vi "odor manifold config to csv (top level vi).vi"() -> ()   [LabVIEW 2021]
uses:
  type-defs/odor and manifold config cluster (type def).ctl
  type-defs/manifold configuration cluster array (type def).ctl
  type-defs/manifold configuration cluster (type def).ctl
  type-defs/manifold selection.ctl
  type-defs/single port single odor cluster.ctl
  type-defs/port number (type def).ctl
  type-defs/odor selection (type def).ctl
  type-defs/odor color (type def).ctl
  type-defs/odor description array (type def).ctl
  type-defs/odor info cluster (type def).ctl
panel:
  out "csv lines out":string[](array[string])
  in  "interactive? (T)":bool=TRUE
  in  "odor manifold config in (none)":T1
  out "error out":errorcluster
  in  "error in (no error)":errorcluster
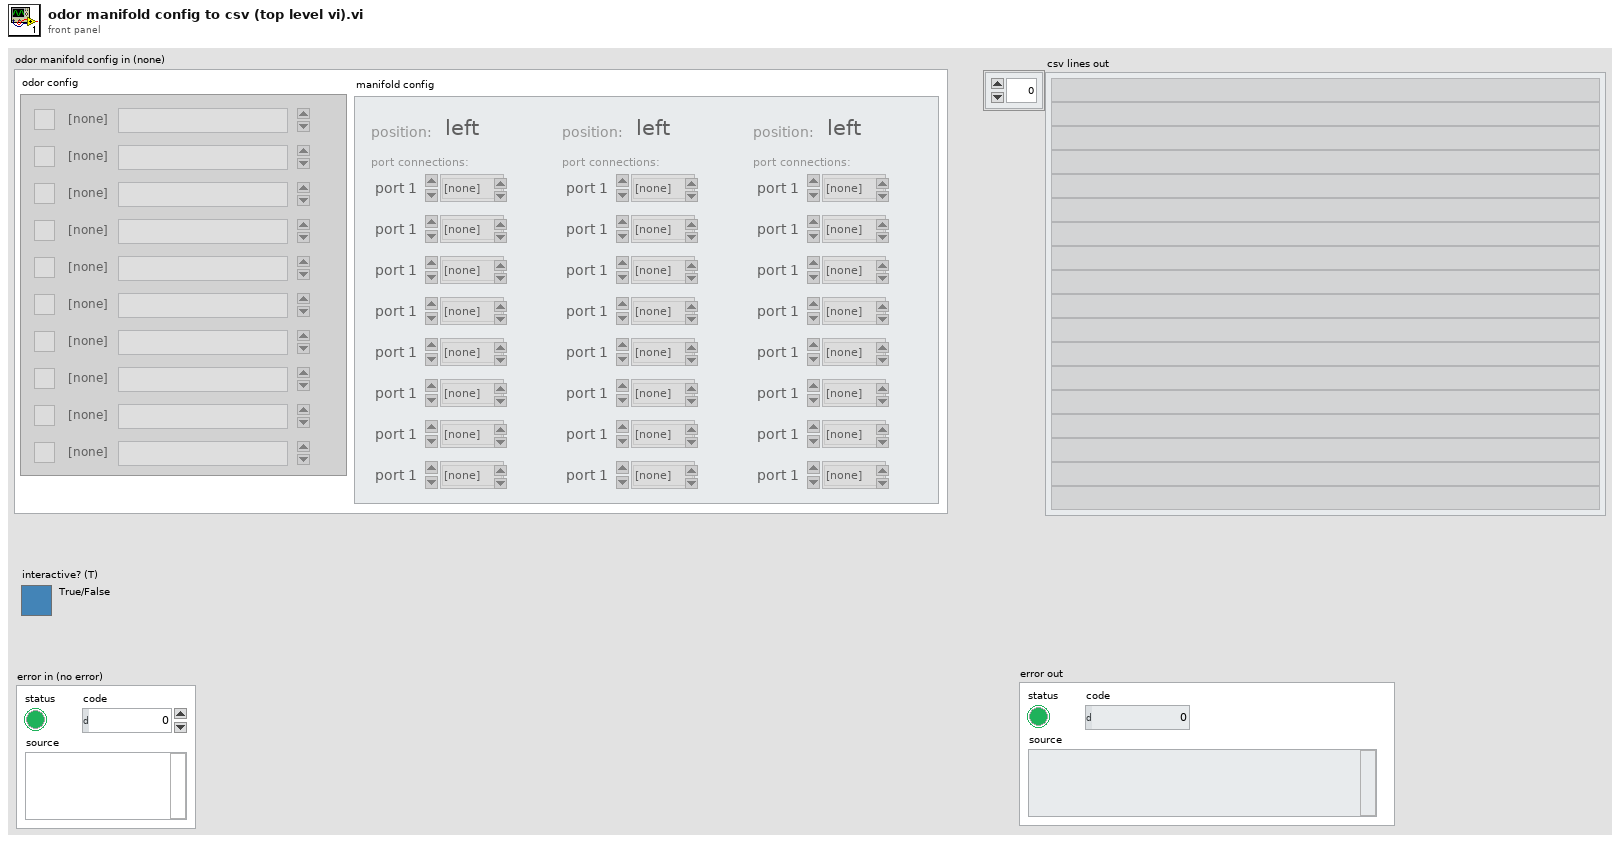
[diagram p1: front panel]
types:
  T1 = typedef "odor and manifold config cluster (type def).ctl" = cluster{"manifold config":T2, "odor config":T9}
  T2 = typedef "manifold configuration cluster array (type def).ctl" = T3[]
  T3 = typedef "manifold configuration cluster (type def).ctl" = cluster{"position:":T4, "port connections:":T5[]}
  T4 = typedef "manifold selection.ctl" = enum16{"left", "middle", "right"}
  T5 = typedef "single port single odor cluster.ctl" = cluster{"port number":T6, "connected odor":T7, "error":bool, "odor color":T8}
  T6 = typedef "port number (type def).ctl" = enum16{"port 1", "port 2", "port 3", "port 4", "port 5", "port 6", "port 7", "port 8"}
  T7 = typedef "odor selection (type def).ctl" = enum16{"[none]", "odor 1", "odor 2", "odor 3", "odor 4", "odor 5", "odor 6", "odor 7", "odor 8", "odor 9", "odor 10"}
  T8 = typedef "odor color (type def).ctl" = u16
  T9 = typedef "odor description array (type def).ctl" = T10[]
  T10 = typedef "odor info cluster (type def).ctl" = cluster{"odor channel":T7, "odor description":string, "odor color":T8, "odor channel active":bool}
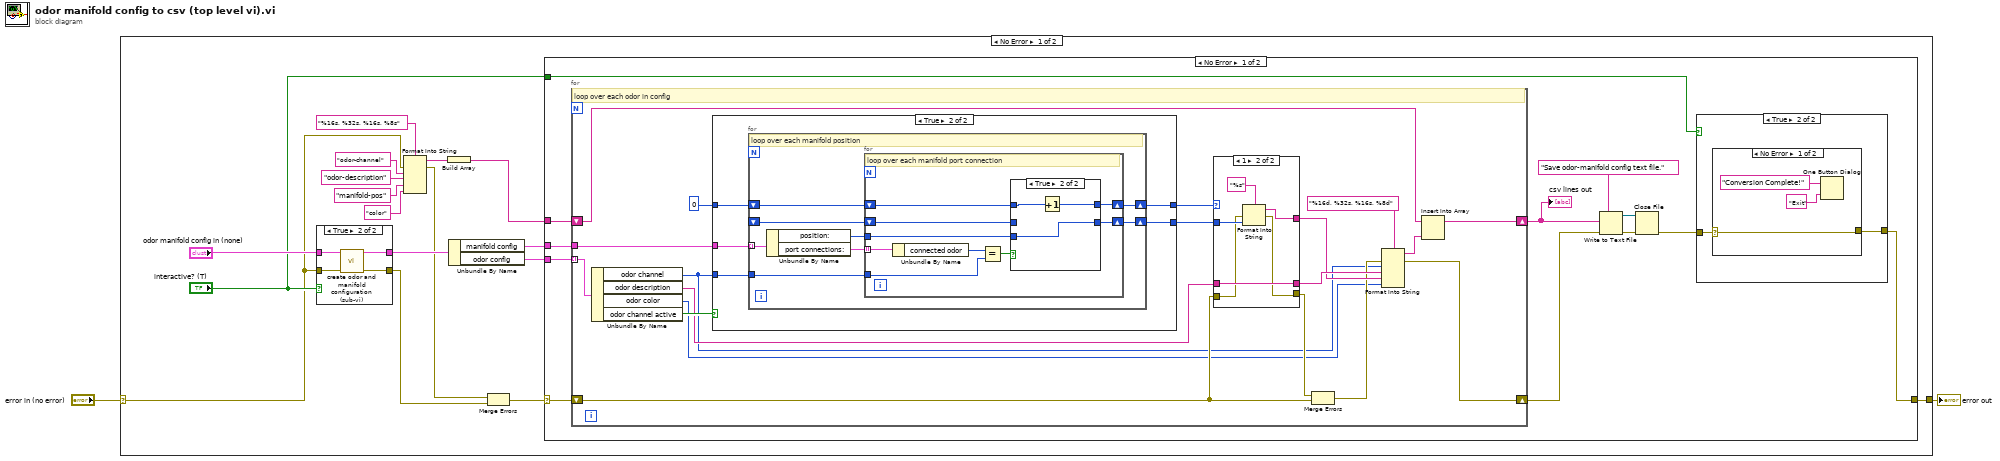
[diagram p0: block diagram]
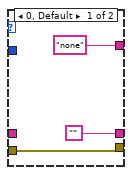
[diagram p5: hidden frame]
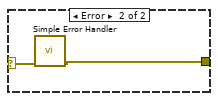
[diagram p7: hidden frame]
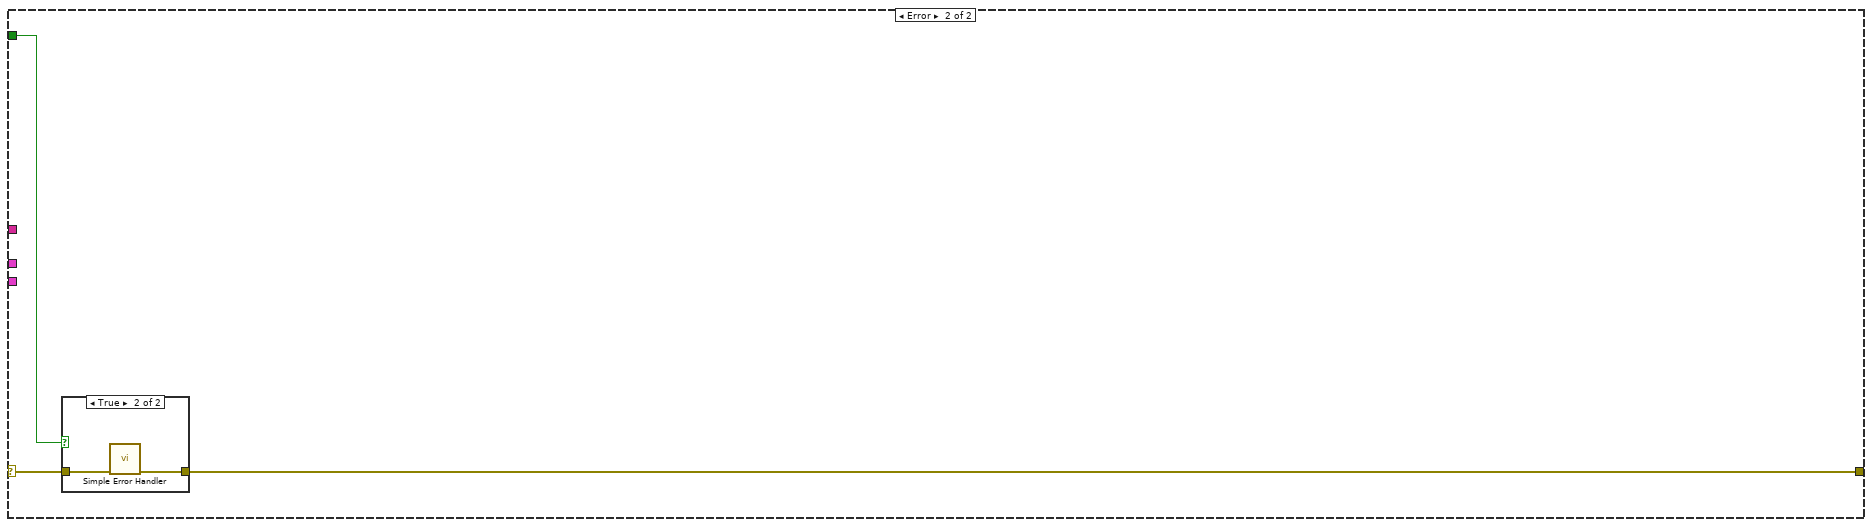
[diagram p8: hidden frame]
diagram:
  n1 = case shown="No Error" "error in (no error)" {
    selector: "error in (no error)" -> [w4 w108]
    tunnel: [w7 w108] -> w1
    frame No Error {
      n2 = case shown="True" "interactive? (T)" {
        tunnel: [w20 w25] -> w11
        tunnel: w4 -> [w21 w24]
        tunnel: [w21 w23] -> w8
        tunnel: "odor manifold config in (none)" -> [w20 w22]
        frame False {
        }
        frame True {
          n3 = call "create odor and manifold configuration (sub-vi).vi"("error in (no error)"=w24, "initial odor and manifold config (none)"=w22) -> ("error out"=w23:errorcluster, "odor and manifold config out"=w25:T1)  [unwired: 7 in, 1 out]
        }
      }
      n4 = Format Into String(format string="%16s, %32s, %16s, %8s", error in=w4, "odor-channel" ("input 1"), "odor-description" ("input 2"), "manifold-pos" ("input 3"), "color" ("input 4")) -> (resulting string=w16:string, error out=w9:errorcluster)  [unwired: 1 in]
      n5 = Build Array(w16) -> (w15:string[])
      n6 = Unbundle By Name(w11) -> ("manifold config"=w18:T2, "odor config"=w19:T9)
      n7 = Merge Errors(w9, w8) -> (w10:errorcluster)
      n8 = case shown="No Error" w10 {
        selector: w10 -> [w29 w104]
        tunnel: w19 -> [w37 _]
        tunnel: w18 -> [w36 _]
        tunnel: w15 -> [w35 _]
        tunnel: [w27 w103] -> w7
        tunnel: "interactive? (T)" -> [w26 w102]
        frame No Error {
          n9 = for {
            tunnel: w37 -> [w55] mode=indexing
            tunnel: w36 -> [w56]
            shift-right: [w46] -> w33
            shift-left: w35 -> [w45]
            shift-right: [w42] -> w30
            shift-left: w29 -> [w41]
            # "loop over each odor in config"
            n10 = Unbundle By Name(w55) -> ("odor channel"=w38:T7, "odor description"=w51:string, "odor color"=w39:T8, "odor channel active"=w54:bool)
            n11 = case shown="True" w54 {
              tunnel: w56 -> [_ w62]
              tunnel: w38 -> [_ w61]
              tunnel: [w57 w60] -> w53
              tunnel: [_ w59] -> w52
              tunnel: 0 -> [w57 w58]
              frame False {
              }
              frame True {
                n12 = for {
                  tunnel: w62 -> [w70] mode=indexing
                  tunnel: w61 -> [w68]
                  shift-right: [w66] -> w59
                  shift-left: _ -> [w65]
                  shift-right: [w63] -> w60
                  shift-left: w58 -> [w64]
                  # "loop over each manifold position"
                  n13 = Unbundle By Name(w70) -> ("position:"=w67:T4, "port connections:"=w69:T5[])
                  n14 = for {
                    tunnel: w69 -> [w79] mode=indexing
                    tunnel: w68 -> [w76]
                    tunnel: w67 -> [w75]
                    shift-right: [w74] -> w66
                    shift-left: w65 -> [w73]
                    shift-right: [w71] -> w63
                    shift-left: w64 -> [w72]
                    # "loop over each manifold port connection"
                    n15 = Unbundle By Name(w79) -> ("connected odor"=w78:T7)
                    n16 = Equal?(x=w78, y=w76) -> (x = y?=w77:bool)
                    n17 = case shown="True" w77 {
                      tunnel: w75 -> [_ w84]
                      tunnel: [w81 w84] -> w74
                      tunnel: w73 -> [w81 _]
                      tunnel: w72 -> [w80 w83]
                      tunnel: [w80 w82] -> w71
                      frame False {
                      }
                      frame True {
                        n18 = Increment(x=w83) -> (x+1=w82:i32)
                      }
                    }
                  }
                }
              }
            }
            n19 = case shown="1" w53 {
              tunnel: w52 -> [_ w91]
              tunnel: w51 -> [_ w93]
              tunnel: ["none" w90] -> w48
              tunnel: ["" w93] -> w49
              tunnel: [w85 w89] -> w44
              tunnel: w41 -> [w85 w88]
              frame 0, Default {
              }
              frame 1 {
                n20 = Format Into String(format string="%s", error in=w88, w91) -> (resulting string=w90:string, error out=w89:errorcluster)  [unwired: 1 in]
              }
            }
            n21 = Merge Errors(w44, w41) -> (w43:errorcluster)
            n22 = Format Into String(format string="%16d, %32s, %16s, %8d", error in=w43, w38, w49, w48, w39) -> (resulting string=w47:string, error out=w42:errorcluster)  [unwired: 1 in]
            n23 = Insert Into Array(array=w45, new element=w47) -> (w46:string[])  [unwired: 1 in]
          }
          "csv lines out" <- w33
          n24 = Write to Text File(prompt (Choose or enter file path)="Save odor-manifold config text file." ("prompt"), text=w33, error in=w30) -> (refnum out=w31:refnum<file>, error out=w32:errorcluster)  [unwired: 1 in, 1 out]
          n25 = Close File(refnum=w31, error in=w32) -> (error out=w28:errorcluster)  [unwired: 1 out]
          n26 = case shown="True" w26 {
            tunnel: w28 -> [w94 w96]
            tunnel: [w94 w95] -> w27
            frame False {
            }
            frame True {
              n27 = case shown="No Error" w96 {
                selector: w96 -> [w97 w101]
                tunnel: [w97 w100] -> w95
                frame No Error {
                  n28 = One Button Dialog(message="Conversion Complete!", button name ("OK")="Exit") -> ()  [unwired: 1 out]
                }
                frame Error {
                  n29 = call <vilib>:"Simple Error Handler.vi"("error in (no error)"=w101) -> ("error out"=w100:errorcluster)  [unwired: 4 in, 4 out]
                }
              }
            }
          }
        }
        frame Error {
          n30 = case shown="True" w102 {
            tunnel: w104 -> [w105 w107]
            tunnel: [w105 w106] -> w103
            frame False {
            }
            frame True {
              n31 = call <vilib>:"Simple Error Handler.vi"("error in (no error)"=w107) -> ("error out"=w106:errorcluster)  [unwired: 4 in, 4 out]
            }
          }
        }
      }
    }
    frame Error {
    }
  }
  "error out" <- w1
